vi "getSerialNumber.vi"(8 "error in":errorcluster, 11 "connection ID":refnum<k5>) -> (0 "error out":errorcluster, 2 "sn out":string, 3 "connection ID":refnum<k5>)   [LabVIEW 2019]
panel:
  in  "Get Command":string="com.attocube.system.getSerialNumber"
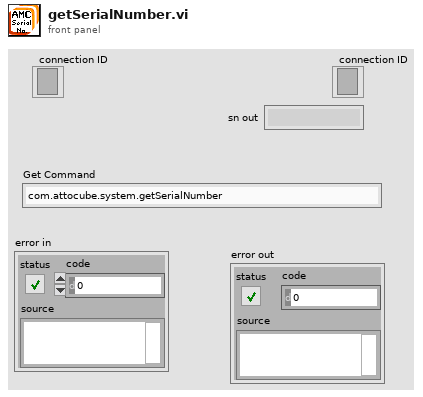
[diagram p1: front panel]
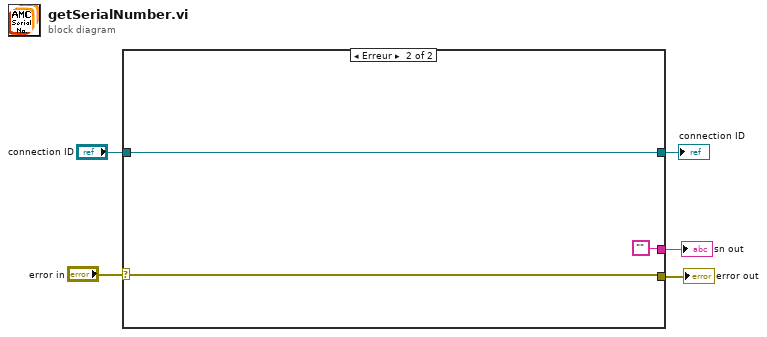
[diagram p0: block diagram]
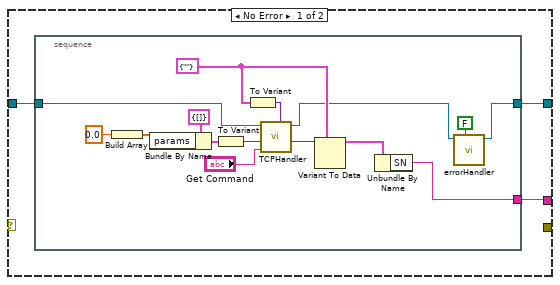
[diagram p2: hidden frame]
diagram:
  n1 = case shown="Erreur" "error in" {
    selector: "error in" -> [_ w26]
    tunnel: [_ w26] -> w5
    tunnel: [w8 ""] -> w4
    tunnel: [w7 w25] -> w3
    tunnel: "connection ID" -> [w6 w25]
    frame No Error {
      n2 = stacked-sequence {
        tunnel: [w9] -> w7
        tunnel: w6 -> [w16]
        tunnel: [w13] -> w8
        frame #0 {
          w14 = cluster{"SN":string} {"SN"=""} ("input cluster")
          n3 = Build Array(0.0 ("element")) -> (w20:dbl[])
          n4 = Bundle By Name(cluster=cluster{"params":i32[]} {"params"=[]} ("input cluster"), "params"=w20) -> (w21:cluster{"params":i32[]})
          n5 = To Variant(anything=w21) -> (Variant=w22:variant)
          n6 = To Variant(anything=w14) -> (Variant=w15:variant)
          n7 = call "TCPHandler.vi"("result Types"=w15, "method"="Get Command", "params"=w22, "connection ID"=w16) -> ("result"=w18:variant, "connection ID"=w10:refnum<k5>)  [unwired: 5 in, 1 out]
          n8 = Variant To Data(type=w14, Variant=w18) -> (data=w23:cluster{"SN":string})  [unwired: 1 in, 1 out]
          n9 = Unbundle By Name(w23) -> ("SN"=w13:string)
          n10 = call "errorHandler.vi"("show popup"=FALSE, "connection ID"=w10) -> ("connection ID"=w9:refnum<k5>)  [unwired: 8 in, 1 out]
        }
      }
    }
    frame Error {
    }
  }
  "error out" <- w5
  "sn out" <- w4
  "connection ID" <- w3
